vi "WFGenA05Bipolar.vi"(1 "Param 0: Inactive":dbl, 2 "Param 1: Inactive":dbl, 3 "Param 2: Inactive":dbl, 4 "Param 3: Inactive":dbl, 5 "error in (no error)":errorcluster, 8 "WFParameters":T2={"Fs (Hz)"=100000.0, "Amp (V)"=1.0, "Ramp (s)"=0.005, "Dur (s)"=0.25} {"Dur (s)" min=0.0 format="%#_4g"; "Ramp (s)" min=0.0; "Fs (Hz)" min=0.0}, 10 "WFRepetitions":T1={"Del (s)"=0.0, "Int (s)"=0.0, "N"=1} {"Int (s)" min=0.0 format="%#_4g"; "Del (s)" min=0.0 format="%#_4f"}) -> (14 "Waveform Out":waveform(dbl), 19 "error out":errorcluster)   [LabVIEW 2013]
uses:
  WFParameters.ctl
  WFRepetitions.ctl
  util/impl/WFComposeA.vi
panel:
  out "Waveform Graph":waveform(dbl)(graph)
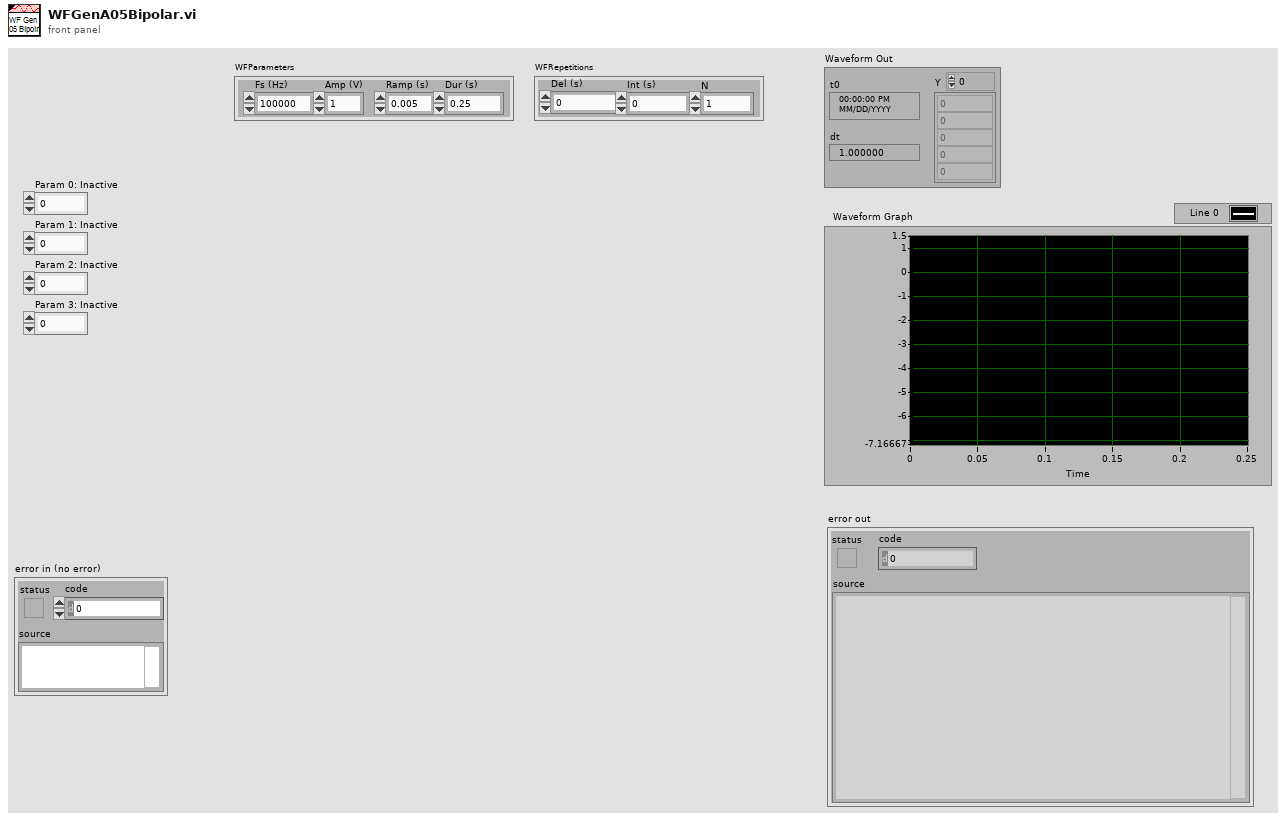
[diagram p1: front panel]
types:
  T1 = typedef "WFRepetitions.ctl" = cluster{"Del (s)":dbl, "Int (s)":dbl, "N":i32}
  T2 = typedef "WFParameters.ctl" = cluster{"Fs (Hz)":dbl, "Amp (V)":dbl, "Ramp (s)":dbl, "Dur (s)":dbl}
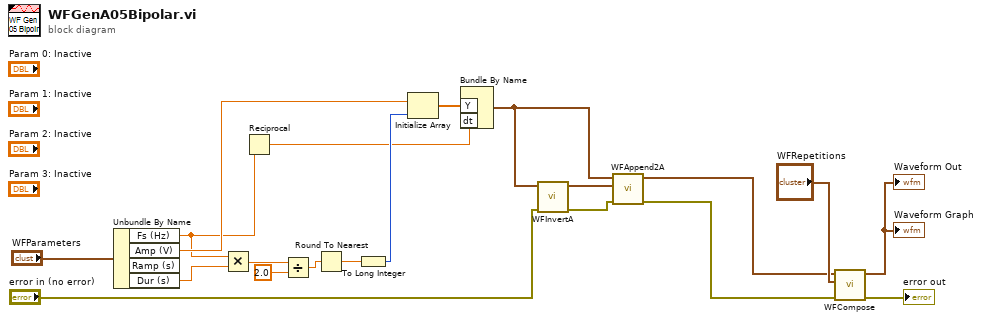
[diagram p0: block diagram]
diagram:
  n1 = Unbundle By Name("WFParameters") -> ("Fs (Hz)"=w10:dbl, "Amp (V)"=w15:dbl, "Dur (s)"=w17:dbl)  [unwired: 1 out]
  n2 = Multiply(x=w10, y=w17) -> (x*y=w9:dbl)
  n3 = Reciprocal(x=w10) -> (1/x=w11:dbl)
  n4 = Divide(x=w9, y=2.0) -> (x/y=w7:dbl)
  n5 = Round To Nearest(number=w7) -> (nearest integer value=w12:dbl)
  n6 = To Long Integer(number=w12) -> (32bit integer=w16:i32)
  n7 = Initialize Array(w15, w16) -> (w14:dbl[])
  n8 = Bundle By Name("Y"=w14, "dt"=w11) -> (w5:waveform(dbl))  [unwired: 1 in]
  n9 = call "WFInvertA.vi"("error in (no error)"="error in (no error)", "Waveform In"=w5) -> ("error out"=w2:errorcluster, "Waveform Out"=w6:waveform(dbl))  [unwired: 4 in]
  n10 = call "WFAppend2A.vi"("error in (no error)"=w2, "Waveform In 2"=w6, "Waveform In"=w5) -> ("error out"=w3:errorcluster, "Waveform Out"=w4:waveform(dbl))  [unwired: 3 in]
  n11 = call-poly "WFCompose.vi"("error in (no error)"=w3, "WFRepetitions"="WFRepetitions", "Waveform In"=w4) -> ("error out"=→"error out":errorcluster, "Analog Waveform Out"=→"Waveform Graph" →"Waveform Out":waveform(dbl))  [unwired: 7 in]
